vi "Log Data DBL.vi"(7 "Time Stamp":timestamp format="%<%x %.3X>T", 8 "error in":errorcluster, 9 "Data":dbl, 10 "Ident":string, 11 "Series Actor in":refnum<class "Series Actor.lvclass">) -> (0 "error out":errorcluster, 3 "Series Actor out":refnum<class "Series Actor.lvclass">)   [LabVIEW 2023, in "Series Actor.lvlib" / "Series Actor.lvclass"]
uses:
  Series Actor.lvclass
  Series Actor.lvclass/Series Actor.ctl
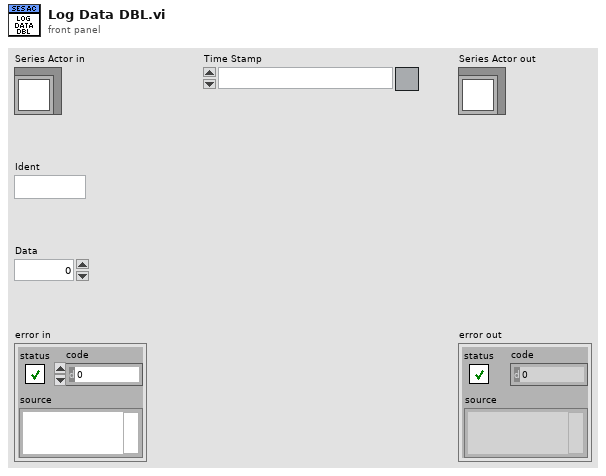
[diagram p1: front panel]
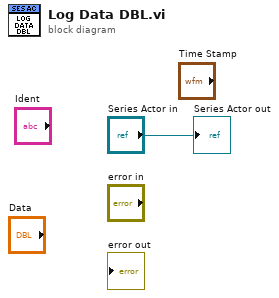
[diagram p0: block diagram]
diagram:
  "Series Actor out" <- "Series Actor in"
